vi "queue.vi"() -> ()   [LabVIEW 2020]
doc: "This VI creates two queues to pass data between parallel loops. Queues are most useful when you need to send data from one or more data sources to one data sink with no potential loss of data."
panel:
  in  "milliseconds to wait 2":u32=200
  in  "milliseconds to wait":u32=100
  out "Data 2":i32(graph)
  out "Data 1":i32(graph)
  in  "Stop":bool
  # "Overview: Demonstrates the use of the Queue functions to pass data between parallel loops.\nInstructions:\nRun the VI."
  # "The data generated by Loop 1 on the diagram is passed to Loop 2 through a queue. The stop condition is also monitored in Loop 1 and sent to Loop 2 in a queue."
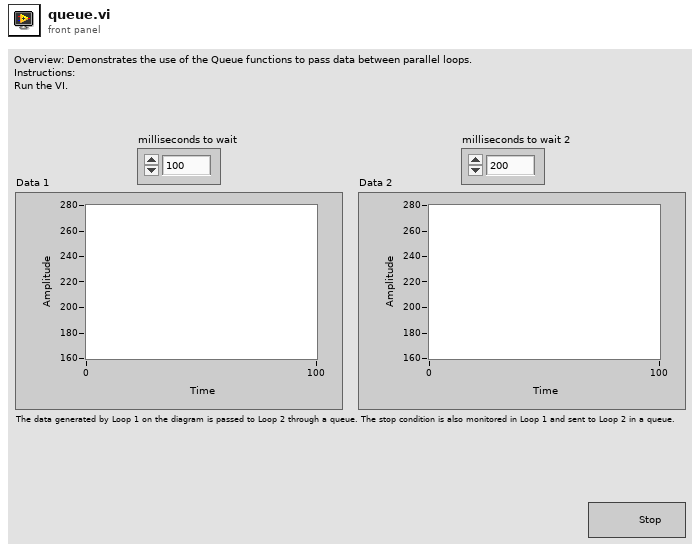
[diagram p1: front panel]
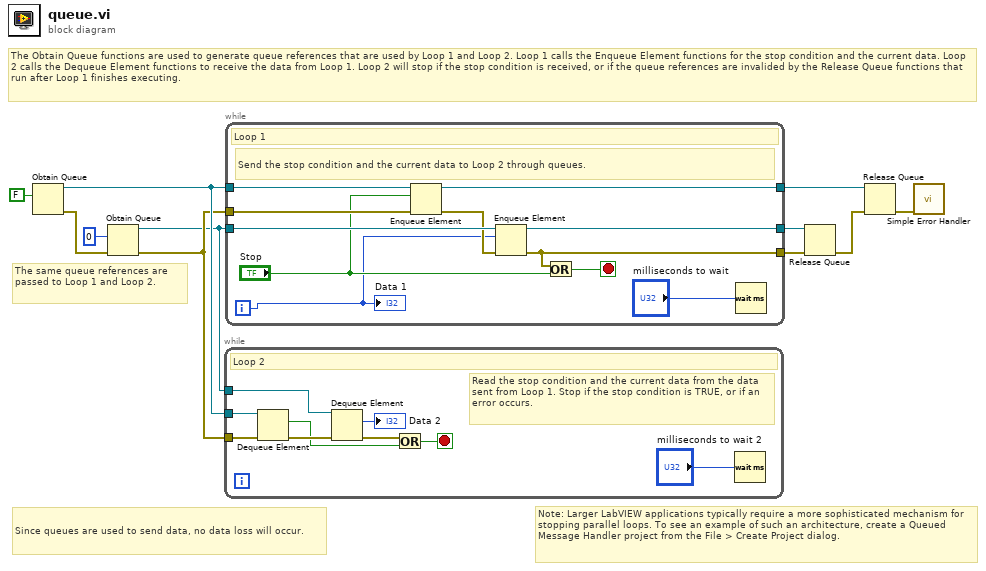
[diagram p0: block diagram]
diagram:
  # "Since queues are used to send data, no data loss will occur."
  # "Note: Larger LabVIEW applications typically require a more sophisticated mechanism for stopping parallel loops. To see an example of such an architecture, create a Queued Message Handler project from the File > Create Project dialog."
  # "The same queue references are passed to Loop 1 and Loop 2."
  # "The Obtain Queue functions are used to generate queue references that are used by Loop 1 and Loop 2. Loop 1 calls the Enqueue Element functions for the stop condition and the current data. Loop 2 calls the Dequeue Element functions to receive the data from Loop 1. Loop 2 will stop if the stop condition is received, or if the queue references are invalided by the Release Queue functions that run after Loop 1 finishes executing."
  n1 = Obtain Queue(element data type=FALSE) -> (queue out=w11:refnum<queue>, error out=w9:errorcluster)  [unwired: 4 in, 1 out]
  n2 = Obtain Queue(element data type=0, error in (no error)=w9) -> (queue out=w1:refnum<queue>, error out=w2:errorcluster)  [unwired: 3 in, 1 out]
  n3 = while {
    tunnel: w11 -> [w19]
    tunnel: w2 -> [w20]
    tunnel: w1 -> [w17]
    stop <- w13 stop-if-true
    # "Read the stop condition and the current data from the data sent from Loop 1. Stop if the stop condition is TRUE, or if an error occurs."
    # "Loop 2"
    n4 = Dequeue Element(queue=w19, error in (no error)=w20) -> (element=w14:bool, error out=w18:errorcluster)  [unwired: 1 in, 2 out]
    n5 = Dequeue Element(queue=w17, error in (no error)=w18) -> (element=→"Data 2":i32, error out=w15:errorcluster)  [unwired: 1 in, 2 out]
    n6 = Or(x=w15, y=w14) -> (x .or. y?=w13:bool)
    n7 = Wait (ms)(milliseconds to wait="milliseconds to wait 2") -> ()  [unwired: 1 out]
  }
  n8 = while {
    tunnel: w11 -> [w30]
    tunnel: w2 -> [w29]
    tunnel: [w28] -> w4
    tunnel: w1 -> [w27]
    tunnel: [w25] -> w6
    tunnel: [w24] -> w7
    i -> [w21]
    stop <- w22 stop-if-true
    # "Send the stop condition and the current data to Loop 2 through queues."
    # "Loop 1"
    n9 = Enqueue Element(queue=w30, element="Stop", error in (no error)=w29) -> (queue out=w28:refnum<queue>, error out=w26:errorcluster)  [unwired: 1 in, 1 out]
    n10 = Enqueue Element(queue=w27, element=w21, error in (no error)=w26) -> (queue out=w25:refnum<queue>, error out=w24:errorcluster)  [unwired: 1 in, 1 out]
    n11 = Or(x=w24, y="Stop") -> (x .or. y?=w22:bool)
    n12 = Wait (ms)(milliseconds to wait="milliseconds to wait") -> ()  [unwired: 1 out]
    "Data 1" <- w21
  }
  n13 = Release Queue(queue=w6, error in (no error)=w7) -> (error out=w5:errorcluster)  [unwired: 1 in, 2 out]
  n14 = Release Queue(queue=w4, error in (no error)=w5) -> (error out=w3:errorcluster)  [unwired: 1 in, 2 out]
  n15 = call <vilib>:"Simple Error Handler.vi"("error in (no error)"=w3) -> ()  [unwired: 4 in, 5 out]
